vi "Destroy.vi"(8 "error in (no error)":errorcluster, 11 "Excel in":refnum<class "Excel.lvclass">) -> (0 "error out":errorcluster)   [LabVIEW 2016, in "Excel.lvclass"]
doc: "Destroys an Excel object releasing all references used for interfacing with Excel."
uses:
  Excel.lvclass
  Excel.lvclass/Excel.ctl
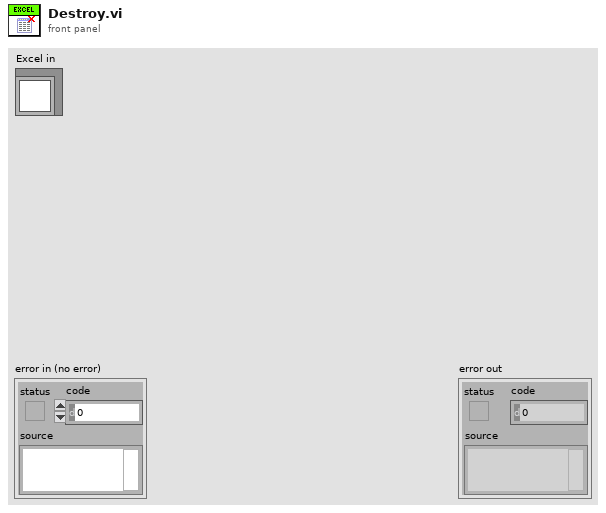
[diagram p1: front panel]
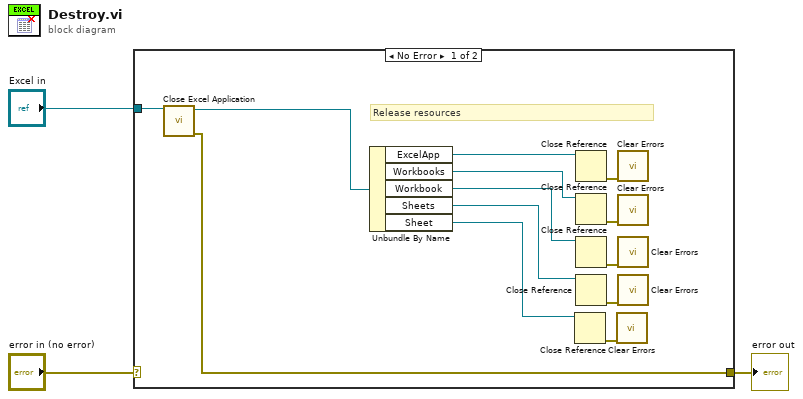
[diagram p0: block diagram]
diagram:
  n1 = case shown="No Error" "error in (no error)" {
    selector: "error in (no error)" -> [_ w17]
    tunnel: [w4 w17] -> w2
    tunnel: "Excel in" -> [w6 _]
    frame No Error {
      # "Release resources"
      n2 = call "Close Excel Application.vi"("Excel in"=w6) -> ("error out"=w4:errorcluster, "Excel out"=w5:refnum<class "Excel.lvclass">)  [unwired: 9 in]
      n3 = Unbundle By Name(w5) -> ("ExcelApp"=w16:refnum<k7>, "Workbooks"=w15:refnum<k7>, "Workbook"=w14:refnum<k7>, "Sheets"=w8:refnum<k7>, "Sheet"=w7:refnum<k7>)
      n4 = Close Reference(reference=w7) -> (error out=w9:errorcluster)  [unwired: 1 in]
      n5 = Close Reference(reference=w16) -> (error out=w13:errorcluster)  [unwired: 1 in]
      n6 = Close Reference(reference=w15) -> (error out=w12:errorcluster)  [unwired: 1 in]
      n7 = Close Reference(reference=w14) -> (error out=w11:errorcluster)  [unwired: 1 in]
      n8 = Close Reference(reference=w8) -> (error out=w10:errorcluster)  [unwired: 1 in]
      n9 = call <vilib>:"Clear Errors.vi"("error in (no error)"=w9) -> ()  [unwired: 5 in, 2 out]
      n10 = call <vilib>:"Clear Errors.vi"("error in (no error)"=w13) -> ()  [unwired: 5 in, 2 out]
      n11 = call <vilib>:"Clear Errors.vi"("error in (no error)"=w12) -> ()  [unwired: 5 in, 2 out]
      n12 = call <vilib>:"Clear Errors.vi"("error in (no error)"=w11) -> ()  [unwired: 5 in, 2 out]
      n13 = call <vilib>:"Clear Errors.vi"("error in (no error)"=w10) -> ()  [unwired: 5 in, 2 out]
    }
    frame Error {
    }
  }
  "error out" <- w2
